vi "a.vi"(6 "Variant in":variant, 7 "Shift Pressed?":bool, 8 "error in (no error)":errorcluster, 10 "QD Combo Box Ref":refnum<vi>, 11 "QD Launch VI Ref":refnum<vi>) -> (0 "error out":errorcluster, 4 "Variant out":variant)   [LabVIEW 2009]
panel:
  in  "Undo Name":string="Object Creation"
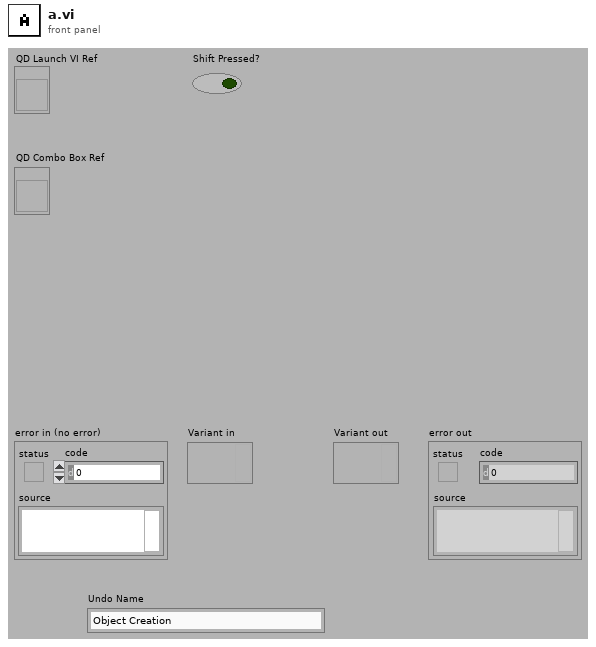
[diagram p1: front panel]
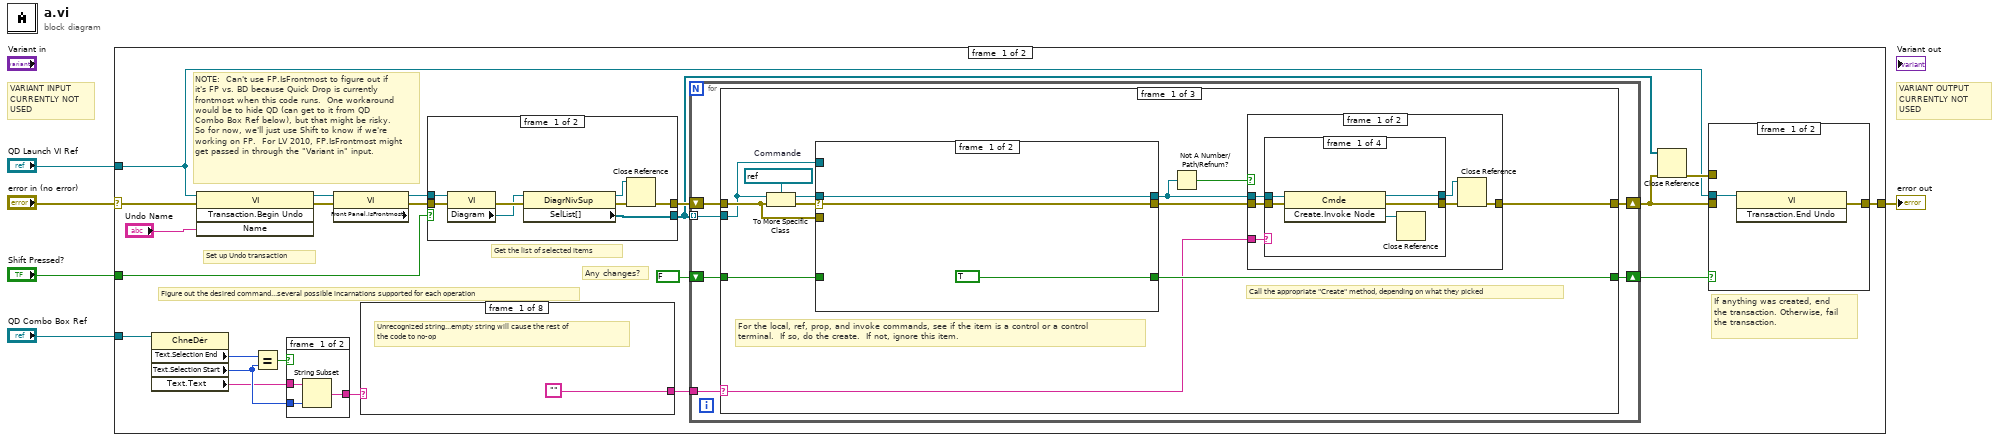
[diagram p0: block diagram]
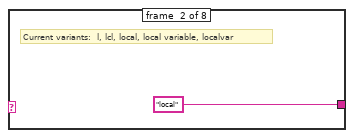
[diagram p2: hidden frame]
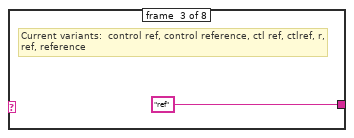
[diagram p3: hidden frame]
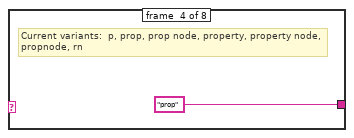
[diagram p4: hidden frame]
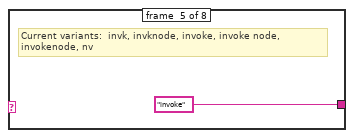
[diagram p5: hidden frame]
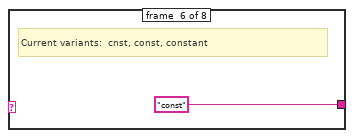
[diagram p6: hidden frame]
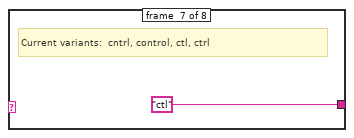
[diagram p7: hidden frame]
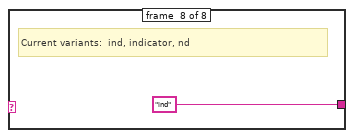
[diagram p8: hidden frame]
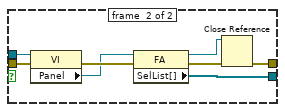
[diagram p10: hidden frame]
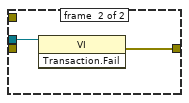
[diagram p11: hidden frame]
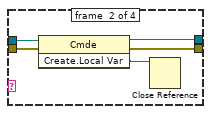
[diagram p12: hidden frame]
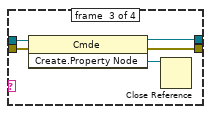
[diagram p13: hidden frame]
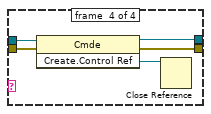
[diagram p14: hidden frame]
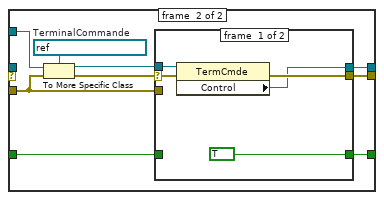
[diagram p16: hidden frame]
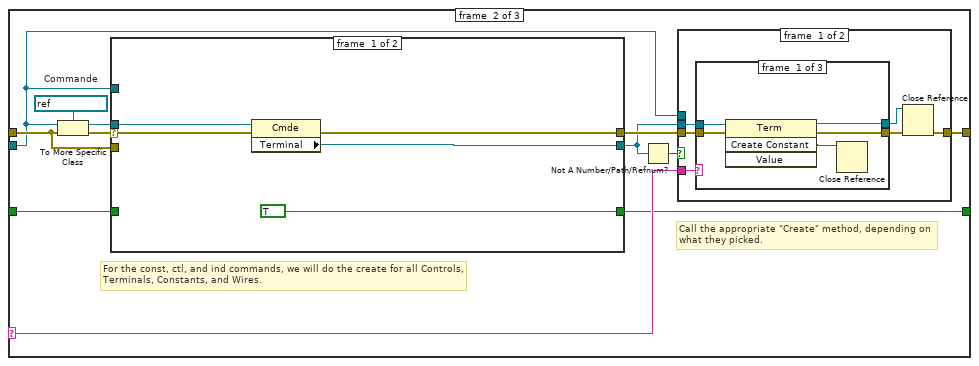
[diagram p18: hidden frame]
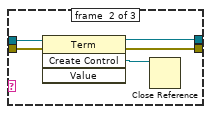
[diagram p19: hidden frame]
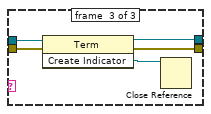
[diagram p20: hidden frame]
diagram:
  # "VARIANT INPUT\nCURRENTLY NOT\nUSED"
  # "VARIANT OUTPUT\nCURRENTLY NOT\nUSED"
  n1 = case shown="Pas d'erreur" "error in (no error)" {
    selector: "error in (no error)" -> [w26 w210]
    tunnel: [w22 w210] -> w4
    tunnel: "Shift Pressed?" -> [w8 _]
    tunnel: "QD Combo Box Ref" -> [w14 _]
    tunnel: "QD Launch VI Ref" -> [w7 _]
    frame #0 {
      # "NOTE:  Can't use FP.IsFrontmost to figure out if it's FP vs. BD because Quick Drop is currently frontmost when this code runs.  One workaround would be to hide QD (can get to it from QD Combo Box Ref below), but that might be risky.  So for now, we'll just use Shift to know if we're working on FP.  For LV 2010, FP.IsFrontmost might get passed in through the \"Variant in\" input."
      # "Figure out the desired command...several possible incarnations supported for each operation"
      # "If anything was created, end the transaction. Otherwise, fail the transaction."
      # "Any changes?"
      # "Get the list of selected items"
      # "Set up Undo transaction"
      n2 = property on="Property Node" class="ChneDér"(reference=w14) -> ("Text.Selection End"=w18:u32, "Text.Selection Start"=w16:u32, "Text.Text"=w15:string)  [unwired: 1 in, 2 out]
      n3 = invoke class="VI" method="Transaction.Begin Undo"(reference=w7, error in=w26, "Name"="Undo Name") -> (reference out=w6:refnum<vi>, error out=w21:errorcluster)  [unwired: 1 in, 2 out]
      n4 = Equal?(x=w18, y=w16) -> (x = y?=w17:bool)
      n5 = case shown="Vrai" w17 {
        tunnel: [w38 w39] -> w13
        tunnel: w16 -> [w37 _]
        tunnel: w15 -> [w36 w39]
        frame #0 {
          n6 = String Subset(string=w36, length (rest)=w37) -> (substring=w38:string)  [unwired: 1 out]
        }
        frame #1 {
        }
      }
      n7 = property class="VI" props=["Front Panel.IsFrontmost"](reference=w6, error in=w21) -> (reference out=w19:refnum<vi>, error out=w20:errorcluster)  [unwired: 1 out]
      n8 = case shown="\"invk\", \"invknode\", \"invoke\", \"invoke node\", \"invokenode\", \"nv\"" w13 {
        tunnel: ["" "local" "ref" "prop" "invoke" "const" "ctl" "ind"] -> w12
        frame #0 {
          # "Unrecognized string...empty string will cause the rest of\nthe code to no-op"
        }
        frame #1 {
          # "Current variants:  l, lcl, local, local variable, localvar"
        }
        frame #2 {
          # "Current variants:  control ref, control reference, ctl ref, ctlref, r, ref, reference"
        }
        frame #3 {
          # "Current variants:  p, prop, prop node, property, property node, propnode, rn"
        }
        frame #4 {
          # "Current variants:  invk, invknode, invoke, invoke node, invokenode, nv"
        }
        frame #5 {
          # "Current variants:  cnst, const, constant"
        }
        frame #6 {
          # "Current variants:  cntrl, control, ctl, ctrl"
        }
        frame #7 {
          # "Current variants:  ind, indicator, nd"
        }
      }
      n9 = case shown="Faux" w8 {
        tunnel: [w45 w53] -> w10
        tunnel: [w44 w52] -> w23
        tunnel: w20 -> [w41 w49]
        tunnel: w19 -> [w40 w48]
        frame #0 {
          n10 = property class="VI"(reference=w40, error in=w41) -> (error out=w47:errorcluster, "Diagram"=w46:refnum<vi>)  [unwired: 1 out]
          n11 = property class="DiagrNivSup"(reference=w46, error in=w47) -> (reference out=w42:refnum<vi>, error out=w43:errorcluster, "SelList[]"=w45:refnum<vi>[])
          n12 = Close Reference(reference=w42, error in (no error)=w43) -> (error out=w44:errorcluster)
        }
        frame #1 {
          n13 = property class="VI"(reference=w48, error in=w49) -> (error out=w55:errorcluster, "Panel"=w54:refnum<vi>)  [unwired: 1 out]
          n14 = property class="FA"(reference=w54, error in=w55) -> (reference out=w50:refnum<vi>, error out=w51:errorcluster, "SelList[]"=w53:refnum<vi>[])
          n15 = Close Reference(reference=w50, error in (no error)=w51) -> (error out=w52:errorcluster)
        }
      }
      n16 = for {
        tunnel: w10 -> [w61] mode=indexing
        shift-right: [w60] -> w11
        shift-left: w23 -> [w65]
        shift-right: [w62] -> w24
        shift-left: FALSE -> [w63]
        tunnel: w12 -> [w64]
        n17 = case shown="\"invoke\", \"local\", \"prop\", \"ref\"" w64 {
          selector: w64 -> [w66 w127 _]
          tunnel: w65 -> [w75 w133 w208]
          tunnel: w61 -> [w71 w125 _]
          tunnel: w63 -> [w73 w131 w209]
          tunnel: [w72 w124 w209] -> w62
          tunnel: [w68 w128 w208] -> w60
          frame #0 {
            w77 = refnum<vi> refnum  # Commande
            # "Call the appropriate \"Create\" method, depending on what they picked"
            # "For the local, ref, prop, and invoke commands, see if the item is a control or a control terminal.  If so, do the create.  If not, ignore this item."
            n18 = To More Specific Class(target class=w77, reference=w71, error in=w75) -> (specific class reference=w74:refnum<vi>, error out=w76:errorcluster)
            n19 = case shown="Erreur" w76 {
              selector: w76 -> [w105 _]
              tunnel: w75 -> [_ w108]
              tunnel: [w107 w109] -> w67
              tunnel: w74 -> [w107 _]
              tunnel: w73 -> [_ w112]
              tunnel: [TRUE w111] -> w72
              tunnel: w71 -> [_ w116]
              tunnel: [w105 w110] -> w69
              frame #0 {
              }
              frame #1 {
                w115 = refnum<vi> refnum  # TerminalCommande
                n20 = To More Specific Class(target class=w115, reference=w116, error in=w108) -> (specific class reference=w113:refnum<vi>, error out=w114:errorcluster)
                n21 = case shown="Pas d'erreur" w114 {
                  selector: w114 -> [w120 _]
                  tunnel: w113 -> [w121 _]
                  tunnel: w112 -> [_ w122]
                  tunnel: [TRUE w122] -> w111
                  tunnel: [w118 w123] -> w110
                  tunnel: [w117 _] -> w109
                  tunnel: w108 -> [_ w123]
                  frame #0 {
                    n22 = property class="TermCmde"(reference=w121, error in=w120) -> (error out=w118:errorcluster, "Control"=w117:refnum<vi>)  [unwired: 1 out]
                  }
                  frame #1 {
                  }
                }
              }
            }
            n23 = Not A Number/Path/Refnum?(number/path/refnum=w67) -> (NaN/Path/Refnum?=w70:bool)
            n24 = case shown="Faux" w70 {
              tunnel: w69 -> [w82 w104]
              tunnel: [w78 w104] -> w68
              tunnel: w67 -> [w81 _]
              tunnel: w66 -> [w83 _]
              frame #0 {
                n25 = case shown="\"local\", Par défaut" w83 {
                  tunnel: w82 -> [w88 w93 w98 w103]
                  tunnel: w81 -> [w87 w92 w97 w102]
                  tunnel: [w86 w91 w96 w101] -> w80
                  tunnel: [w84 w89 w94 w99] -> w79
                  frame #0 {
                    n26 = invoke class="Cmde" method="Create.Invoke Node"(reference=w87, error in=w88) -> (reference out=w84:refnum<vi>, error out=w86:errorcluster, "Create Invoke Node"=w85:refnum<vi>)  [unwired: 1 in]
                    n27 = Close Reference(reference=w85) -> ()  [unwired: 1 in, 1 out]
                  }
                  frame #1 {
                    n28 = invoke class="Cmde" method="Create.Local Var"(reference=w92, error in=w93) -> (reference out=w89:refnum<vi>, error out=w91:errorcluster, "Create Local"=w90:refnum<vi>)  [unwired: 1 in]
                    n29 = Close Reference(reference=w90) -> ()  [unwired: 1 in, 1 out]
                  }
                  frame #2 {
                    n30 = invoke class="Cmde" method="Create.Property Node"(reference=w97, error in=w98) -> (reference out=w94:refnum<vi>, error out=w96:errorcluster, "Create Property Node"=w95:refnum<vi>)  [unwired: 1 in]
                    n31 = Close Reference(reference=w95) -> ()  [unwired: 1 in, 1 out]
                  }
                  frame #3 {
                    n32 = invoke class="Cmde" method="Create.Control Ref"(reference=w102, error in=w103) -> (reference out=w99:refnum<vi>, error out=w101:errorcluster, "Create Control Ref"=w100:refnum<vi>)  [unwired: 1 in]
                    n33 = Close Reference(reference=w100) -> ()  [unwired: 1 in, 1 out]
                  }
                }
                n34 = Close Reference(reference=w79, error in (no error)=w80) -> (error out=w78:errorcluster)
              }
              frame #1 {
              }
            }
          }
          frame #1 {
            w135 = refnum<vi> refnum  # Commande
            # "Call the appropriate \"Create\" method, depending on what they picked."
            # "For the const, ctl, and ind commands, we will do the create for all Controls, Terminals, Constants, and Wires."
            n35 = To More Specific Class(target class=w135, reference=w125, error in=w133) -> (specific class reference=w132:refnum<vi>, error out=w134:errorcluster)
            n36 = case shown="Erreur" w134 {
              selector: w134 -> [w161 _]
              tunnel: w133 -> [_ w165]
              tunnel: w132 -> [w160 _]
              tunnel: w131 -> [_ w168]
              tunnel: [TRUE w167] -> w124
              tunnel: w125 -> [_ w163]
              tunnel: [w159 w166] -> w129
              tunnel: [w158 w164] -> w126
              frame #0 {
                n37 = property class="Cmde"(reference=w160, error in=w161) -> (error out=w159:errorcluster, "Terminal"=w158:refnum<vi>)  [unwired: 1 out]
              }
              frame #1 {
                w171 = refnum<vi> refnum  # Terminal
                n38 = To More Specific Class(target class=w171, reference=w163, error in=w165) -> (specific class reference=w169:refnum<vi>, error out=w170:errorcluster)
                n39 = case shown="Erreur" w170 {
                  selector: w170 -> [w173 _]
                  tunnel: w169 -> [w172 _]
                  tunnel: w168 -> [_ w177]
                  tunnel: [TRUE w176] -> w167
                  tunnel: [w173 w178] -> w166
                  tunnel: w165 -> [_ w181]
                  tunnel: [w172 w179] -> w164
                  tunnel: w163 -> [_ w175]
                  frame #0 {
                  }
                  frame #1 {
                    w183 = refnum<vi> refnum  # Constante
                    n40 = To More Specific Class(target class=w183, reference=w175, error in=w181) -> (specific class reference=w180:refnum<vi>, error out=w182:errorcluster)
                    n41 = case shown="Erreur" w182 {
                      selector: w182 -> [w188 _]
                      tunnel: w181 -> [_ w191]
                      tunnel: w180 -> [w187 _]
                      tunnel: [w186 w192] -> w179
                      tunnel: [w185 w193] -> w178
                      tunnel: w177 -> [_ w190]
                      tunnel: [TRUE w189] -> w176
                      tunnel: w175 -> [_ w197]
                      frame #0 {
                        n42 = property class="Cste"(reference=w187, error in=w188) -> (error out=w185:errorcluster, "Terminal"=w186:refnum<vi>)  [unwired: 1 out]
                      }
                      frame #1 {
                        w196 = refnum<vi> refnum  # Fil de liaison
                        n43 = To More Specific Class(target class=w196, reference=w197, error in=w191) -> (specific class reference=w194:refnum<vi>, error out=w195:errorcluster)
                        n44 = case shown="Pas d'erreur" w195 {
                          selector: w195 -> [w205 _]
                          tunnel: w194 -> [w204 _]
                          tunnel: [w203 w207] -> w193
                          tunnel: [w200 _] -> w192
                          tunnel: w191 -> [_ w207]
                          tunnel: w190 -> [_ w206]
                          tunnel: [TRUE w206] -> w189
                          frame #0 {
                            n45 = property class="Fil"(reference=w204, error in=w205) -> (error out=w203:errorcluster, "Terms[]"=w202:refnum<vi>[])  [unwired: 1 out]
                            n46 = Delete From Array(array=w202, index=0) -> (deleted portion=w200:refnum<vi>, array with subset deleted=w199:refnum<vi>[])  [unwired: 1 in]
                            n47 = Close Reference(reference=w199) -> ()  [unwired: 1 in, 1 out]
                          }
                          frame #1 {
                          }
                        }
                      }
                    }
                  }
                }
              }
            }
            n48 = Not A Number/Path/Refnum?(number/path/refnum=w126) -> (NaN/Path/Refnum?=w130:bool)
            n49 = case shown="Faux" w130 {
              tunnel: w129 -> [w140 w157]
              tunnel: [w136 w157] -> w128
              tunnel: w126 -> [w139 _]
              tunnel: w127 -> [w141 _]
              tunnel: w125 -> [_ _]
              frame #0 {
                n50 = case shown="\"const\", Par défaut" w141 {
                  tunnel: w140 -> [w146 w151 w156]
                  tunnel: w139 -> [w145 w150 w155]
                  tunnel: [w144 w149 w154] -> w138
                  tunnel: [w142 w147 w152] -> w137
                  frame #0 {
                    n51 = invoke class="Term" method="Create Constant"(reference=w145, error in=w146) -> (reference out=w142:refnum<vi>, error out=w144:errorcluster, "Create Constant"=w143:refnum<vi>)  [unwired: 2 in, 1 out]
                    n52 = Close Reference(reference=w143) -> ()  [unwired: 1 in, 1 out]
                  }
                  frame #1 {
                    n53 = invoke class="Term" method="Create Control"(reference=w150, error in=w151) -> (reference out=w147:refnum<vi>, error out=w149:errorcluster, "Create Control"=w148:refnum<vi>)  [unwired: 2 in, 1 out]
                    n54 = Close Reference(reference=w148) -> ()  [unwired: 1 in, 1 out]
                  }
                  frame #2 {
                    n55 = invoke class="Term" method="Create Indicator"(reference=w155, error in=w156) -> (reference out=w152:refnum<vi>, error out=w154:errorcluster, "Create Indicator"=w153:refnum<vi>)  [unwired: 1 in]
                    n56 = Close Reference(reference=w153) -> ()  [unwired: 1 in, 1 out]
                  }
                }
                n57 = Close Reference(reference=w137, error in (no error)=w138) -> (error out=w136:errorcluster)
              }
              frame #1 {
              }
            }
          }
          frame #2 {
            # "Unrecognized command...do nothing"
          }
        }
      }
      n58 = Close Reference(reference=w10, error in (no error)=w11) -> (error out=w9:errorcluster)
      n59 = case shown="Vrai" w24 {
        tunnel: w11 -> [_ _]
        tunnel: w7 -> [w56 w58]
        tunnel: [w57 w59] -> w22
        tunnel: w9 -> [_ _]
        frame #0 {
          n60 = invoke class="VI" method="Transaction.End Undo"(reference=w56) -> (error out=w57:errorcluster)  [unwired: 2 in, 2 out]
        }
        frame #1 {
          n61 = invoke class="VI" method="Transaction.Fail"(reference=w58) -> (error out=w59:errorcluster)  [unwired: 2 in, 2 out]
        }
      }
    }
    frame #1 {
    }
  }
  "error out" <- w4
